vi "Actor-Template API.vi"(8 "error in (no error)":errorcluster) -> (0 "error out":errorcluster)   [LabVIEW 2018]
uses:
  Scripting/Interface.lvclass/Interface.ctl
  <vilib>/Utility/error.llb/Clear Errors.vi
  Scripting/Actor.lvclass
  <vilib>/addons/_JKI Toolkits/Caraya/classes/Test/Test.lvclass
  Scripting/Interface.lvclass
  <vilib>/addons/_JKI Toolkits/Caraya/classes/Assert/Assert.lvclass
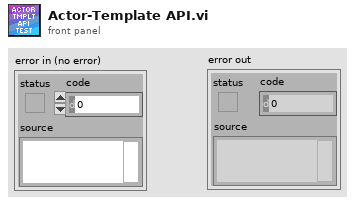
[diagram p1: front panel]
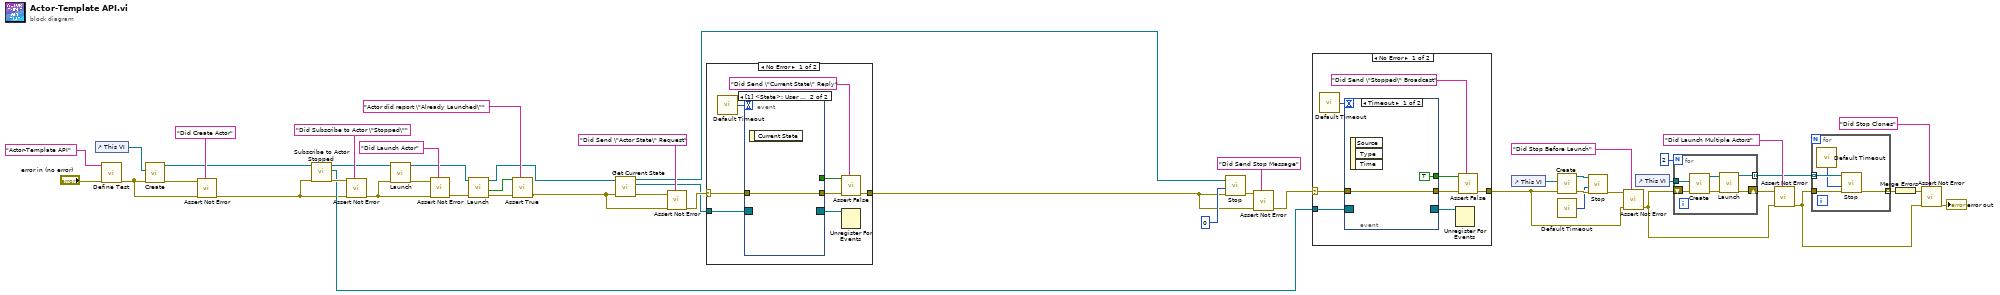
[diagram p0: block diagram]
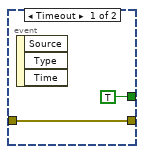
[diagram p2: hidden frame]
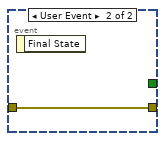
[diagram p4: hidden frame]
diagram:
  n1 = control-ref of="This VI"() -> (w13:refnum<vi>)
  n2 = call <vilib>:"Define Test.vi"("error in (no error)"="error in (no error)", "Label (VI Title)"="Actor-Template API") -> ("error out"=w46:errorcluster)  [unwired: 9 in]
  n3 = call "Create.vi"("error in (no error)"=w46, "Owner"=w13) -> ("error out"=w48:errorcluster, "API out"=w4:refnum<class "Interface.lvclass">)  [unwired: 8 in]
  n4 = call <vilib>:"Assert Not Error.vi"("Label"="Did Create Actor", "error in (no error)"=w46, "Not Error?"=w48) -> ("error out"=w3:errorcluster)  [unwired: 8 in]
  n5 = call "Subscribe to Actor Stopped.vi"("error in (no error)"=w3, "API in"=w4) -> ("error out"=w45:errorcluster, "Actor-Stopped Message"=w34:refnum<event-registration>, "API out"=w43:refnum<class "Interface.lvclass">)  [unwired: 7 in]
  n6 = call <vilib>:"Assert Not Error.vi"("Label"="Did Subscribe to Actor \"Stopped\"", "error in (no error)"=w3, "Not Error?"=w45) -> ("error out"=w41:errorcluster)  [unwired: 8 in]
  n7 = call "Launch.vi"("error in (no error)"=w41, "API in"=w43) -> ("error out"=w42:errorcluster, "API out"=w36:refnum<class "Interface.lvclass">)  [unwired: 7 in, 1 out]
  n8 = call <vilib>:"Assert Not Error.vi"("Label"="Did Launch Actor", "error in (no error)"=w41, "Not Error?"=w42) -> ("error out"=w38:errorcluster)  [unwired: 8 in]
  n9 = call "Launch.vi"("error in (no error)"=w38, "API in"=w36) -> ("error out"=w37:errorcluster, "Already Launched"=w39:bool, "API out"=w10:refnum<class "Interface.lvclass">)  [unwired: 7 in]
  n10 = call <vilib>:"Assert True.vi"("Label"="Actor did report \"Already Launched\"", "error in (no error)"=w37, "True?"=w39) -> ("error out"=w2:errorcluster)  [unwired: 8 in]
  n11 = call "Get Current State.vi"("error in (no error)"=w2, "API In"=w10) -> ("error out"=w9:errorcluster, "State Messages"=w6:refnum<event-registration>, "API out"=w5:refnum<class "Interface.lvclass">)  [unwired: 7 in]
  n12 = call <vilib>:"Assert Not Error.vi"("Label"="Did Send \"Actor State\" Request", "error in (no error)"=w2, "Not Error?"=w9) -> ("error out"=w7:errorcluster)  [unwired: 8 in]
  n13 = case shown="No Error" w7 {
    selector: w7 -> [w56 w62]
    tunnel: w6 -> [w58 _]
    tunnel: [w51 w62] -> w1
    frame No Error {
      n14 = call "Default Timeout.vi"() -> ("Timeout"=w57:i32)
      n15 = event shown="[1] <State>: User Event" {
        selector: w58 -> [_ _]
        dyn-events: [_ _] -> w52
        timeout: w57 -> [_ _]
        tunnel: w56 -> [w59 w61]
        tunnel: [w59 w61] -> w54
        tunnel: [TRUE _] -> w53
        event Timeout {
          n16 = event-data() -> ()  [unwired: 1 in, 3 out]
        }
        event User Event {
          n17 = event-data() -> ()  [unwired: 1 in, 1 out]
        }
      }
      n18 = call <vilib>:"Assert False.vi"("Label"="Did Send \"Current State\" Reply", "error in (no error)"=w54, "False?"=w53) -> ("error out"=w51:errorcluster)  [unwired: 8 in]
      n19 = Unregister For Events(event registration refnum=w52) -> ()  [unwired: 1 in, 1 out]
    }
    frame Error {
    }
  }
  n20 = call "Stop.vi"("error in (no error)"=w1, "Wait for Actor Stop Timeout ms (-1)"=0 ("Wait for Stop Timeout (0 - do not wait)"), "API out"=w5) -> ("error out"=w33:errorcluster)  [unwired: 6 in, 2 out]
  n21 = call <vilib>:"Assert Not Error.vi"("Label"="Did Send Stop Message", "error in (no error)"=w1, "Not Error?"=w33) -> ("error out"=w31:errorcluster)  [unwired: 8 in]
  n22 = case shown="No Error" w31 {
    selector: w31 -> [w68 w74]
    tunnel: w34 -> [w70 _]
    tunnel: [w63 w74] -> w15
    frame No Error {
      n23 = call "Default Timeout.vi"() -> ("Timeout"=w69:i32)
      n24 = event shown="[0] Timeout" {
        selector: w70 -> [_ _]
        dyn-events: [_ _] -> w64
        timeout: w69 -> [_ _]
        tunnel: w68 -> [w71 w73]
        tunnel: [w71 w73] -> w66
        tunnel: [TRUE _] -> w65
        event Timeout {
          n25 = event-data() -> ()  [unwired: 1 in, 3 out]
        }
        event User Event {
          n26 = event-data() -> ()  [unwired: 1 in, 1 out]
        }
      }
      n27 = Unregister For Events(event registration refnum=w64) -> ()  [unwired: 1 in, 1 out]
      n28 = call <vilib>:"Assert False.vi"("Label"="Did Send \"Stopped\" Broadcast", "error in (no error)"=w66, "False?"=w65) -> ("error out"=w63:errorcluster)  [unwired: 8 in]
    }
    frame Error {
    }
  }
  n29 = control-ref of="This VI"() -> (w12:refnum<vi>)
  n30 = call "Create.vi"("error in (no error)"=w15, "Owner"=w12) -> ("error out"=w20:errorcluster, "API out"=w19:refnum<class "Interface.lvclass">)  [unwired: 8 in]
  n31 = call "Default Timeout.vi"() -> ("Timeout"=w18:i32)
  n32 = call "Stop.vi"("error in (no error)"=w20, "Wait for Actor Stop Timeout ms (-1)"=w18, "API out"=w19) -> ("error out"=w16:errorcluster)  [unwired: 6 in, 2 out]
  n33 = call <vilib>:"Assert Not Error.vi"("Label"="Did Stop Before Launch", "error in (no error)"=w15, "Not Error?"=w16) -> ("error out"=w26:errorcluster)  [unwired: 8 in]
  n34 = control-ref of="This VI"() -> (w11:refnum<vi>)
  n35 = for {
    N: 2 -> [_]
    tunnel: [w77] -> w25 mode=indexing
    shift-right: [w76] -> w28
    shift-left: w26 -> [w80]
    tunnel: w11 -> [w75]
    n36 = call "Create.vi"("error in (no error)"=w80, "Owner"=w75) -> ("error out"=w79:errorcluster, "API out"=w78:refnum<class "Interface.lvclass">)  [unwired: 8 in]
    n37 = call "Launch.vi"("error in (no error)"=w79, "API in"=w78) -> ("error out"=w76:errorcluster, "API out"=w77:refnum<class "Interface.lvclass">)  [unwired: 7 in, 1 out]
  }
  n38 = call <vilib>:"Assert Not Error.vi"("Label"="Did Launch Multiple Actors", "error in (no error)"=w26, "Not Error?"=w28) -> ("error out"=w22:errorcluster)  [unwired: 8 in]
  n39 = for {
    tunnel: w25 -> [w84] mode=indexing
    tunnel: w22 -> [w83]
    tunnel: [w81] -> w17 mode=indexing
    n40 = call "Default Timeout.vi"() -> ("Timeout"=w82:i32)
    n41 = call "Stop.vi"("error in (no error)"=w83, "Wait for Actor Stop Timeout ms (-1)"=w82, "API out"=w84) -> ("error out"=w81:errorcluster)  [unwired: 6 in, 2 out]
  }
  n42 = Merge Errors(w17) -> (w24:errorcluster)
  n43 = call <vilib>:"Assert Not Error.vi"("Label"="Did Stop Clones", "error in (no error)"=w22, "Not Error?"=w24) -> ("error out"=→"error out":errorcluster)  [unwired: 8 in]
